vi "timing_and_saving_subVI.vi"(0 "stop":bool, 1 "hrs":dbl, 2 "Data saving":T1(ring), 5 "Auto stop after":bool, 7 "elapsed minutes":dbl, 9 "time to start saving?":bool, 11 "sequence finished":bool, 12 "elapsed minutes":dbl, 13 "Run Sequence":bool) -> (4 "STOP EVERYTHING":bool, 6 "currently saving":bool, 10 "save elapsed time":string)   [LabVIEW 2014]
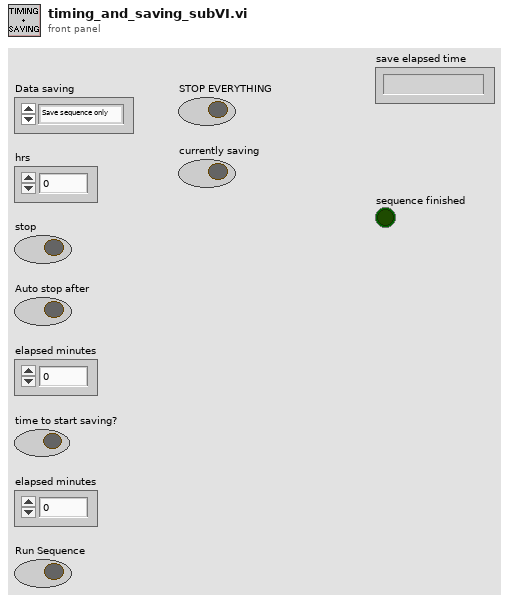
[diagram p1: front panel]
types:
  T1 = enum32{"Save sequence only", " Manually save data"}
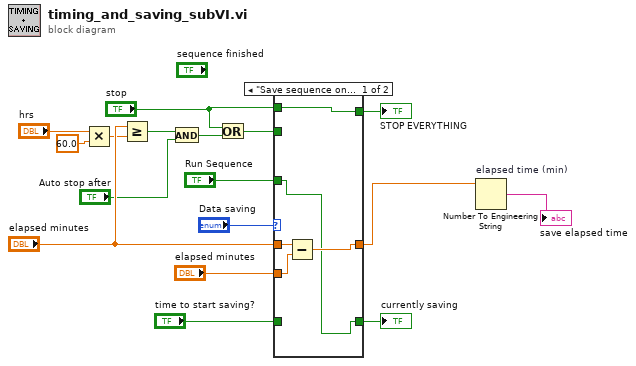
[diagram p0: block diagram]
diagram:
  n1 = Multiply(x="hrs", y=60.0) -> (x*y=w8:dbl)
  n2 = Greater Or Equal?(x="elapsed minutes", y=w8) -> (x >= y?=w3:bool)
  n3 = And(x=w3, y="Auto stop after") -> (x .and. y?=w5:bool)
  n4 = Or(x="stop", y=w5) -> (x .or. y?=w10:bool)
  n5 = case shown="\"Save sequence only\", Default" "Data saving" {
    tunnel: [w18 w25] -> w9
    tunnel: w10 -> [_ w25]
    tunnel: "time to start saving?" -> [_ w24]
    tunnel: [w19 w24] -> w17
    tunnel: "stop" -> [w18 _]
    tunnel: "Run Sequence" -> [w19 _]
    tunnel: "elapsed minutes" -> [w22 w23]
    tunnel: [w20 w23] -> w2
    tunnel: "elapsed minutes" -> [w21 _]
    frame "Save sequence only", Default {
      n6 = Subtract(x=w22, y=w21) -> (x-y=w20:dbl)
    }
    frame " Manually save data" {
    }
  }
  "currently saving" <- w17
  "STOP EVERYTHING" <- w9
  n7 = Number To Engineering String "elapsed time (min)"(4:w2) -> (0:→"save elapsed time":string)  [unwired: 3 in]
